vi "Write Connection String.vi"(8 "error in (no error)":errorcluster, 10 "Connection String":string, 11 "LV-Data.PGSQL in":refnum<class "LV-Data.PGSQL.lvclass">) -> (0 "error out":errorcluster, 3 "LV-Data.PGSQL out":refnum<class "LV-Data.PGSQL.lvclass">)   [LabVIEW 2019, in "LV-Data.PGSQL.lvclass"]
uses:
  LV-Data.PGSQL.lvclass
  LV-Data.PGSQL.lvclass/LV-Data.PGSQL.ctl
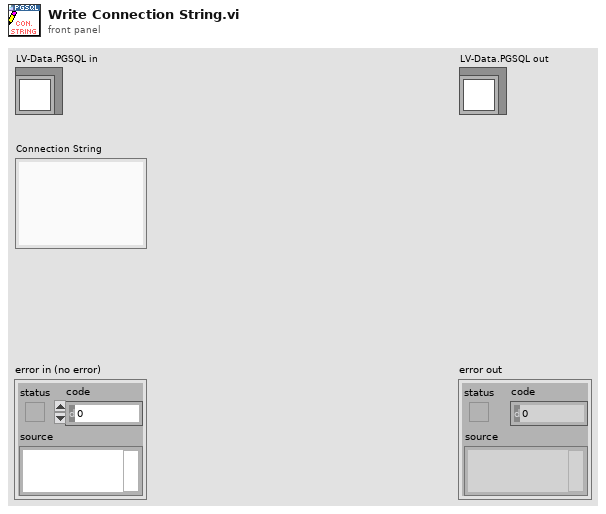
[diagram p1: front panel]
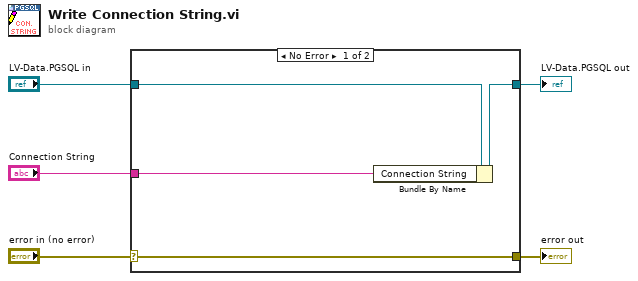
[diagram p0: block diagram]
diagram:
  n1 = case shown="No Error" "error in (no error)" {
    selector: "error in (no error)" -> [w9 w10]
    tunnel: [w9 w10] -> w4
    tunnel: [w7 w11] -> w2
    tunnel: "LV-Data.PGSQL in" -> [w8 w11]
    tunnel: "Connection String" -> [w6 _]
    frame No Error {
      n2 = Bundle By Name(cluster=w8, "Connection String"=w6) -> (w7:refnum<class "LV-Data.PGSQL.lvclass">)
    }
    frame Error {
    }
  }
  "error out" <- w4
  "LV-Data.PGSQL out" <- w2
